vi "Queue Add Events to Back.vi"(0 "Queue In":refnum<queue>, 1 "State Array":cluster{"State":string}[](array[cluster]), 11 "Error In":errorcluster) -> (4 "Queue Out":refnum<queue>, 15 "Error Out":errorcluster)   [LabVIEW 2020]
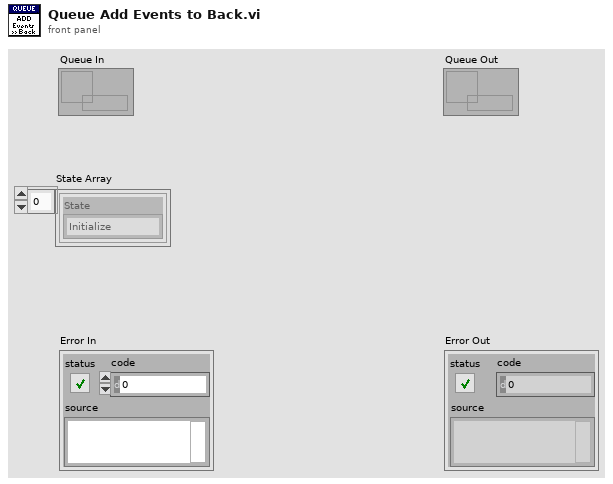
[diagram p1: front panel]
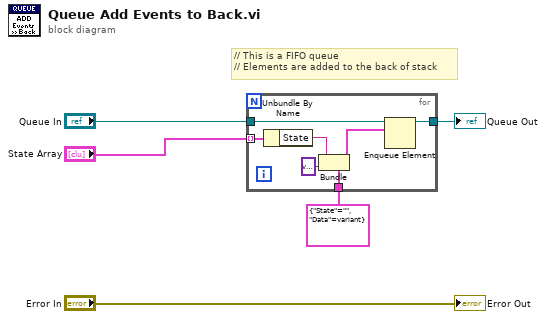
[diagram p0: block diagram]
diagram:
  # "// This is a FIFO queue\n// Elements are added to the back of stack"
  n1 = for {
    tunnel: "State Array" -> [w9] mode=indexing
    tunnel: "Queue In" -> [w12]
    tunnel: [w11] -> w2
    tunnel: cluster{"State":string, "Data":variant} {"State"="", "Data"=variant} ("Cluster") -> [w10]
    n2 = Unbundle By Name(w9) -> ("State"=w8:string)
    n3 = Bundle(cluster=w10, "State"=w8, "Data"=variant) -> (w6:cluster{"State":string, "Data":variant})
    n4 = Enqueue Element(queue=w12, element=w6) -> (queue out=w11:refnum<queue>)  [unwired: 2 in, 2 out]
  }
  "Queue Out" <- w2
  "Error Out" <- "Error In"
